vi "VMI_camera_Set.vi"(8 "error in (no error)":errorcluster, 10 "Camera Settings":T1={"Run Options"=1, "Run Mode"=0, "Attributes"="[NIIMAQ_HEADER]\nType = 2\nVersion = 8\n\n[CAMERA_DATA]\nAcquisitionAttributes::VideoMode = \"640 x 480 Mono 8 60.00 fps\"\nAcquisitionAttributes::OffsetX = \"0\"\nAcquisitionAttributes::OffsetY = \"0\"\nAcquisitionAttributes::Width = \"640\"\nAcquisitionAttributes::Height = \"480\"\nAcquisitionAttributes::Bayer::Algorithm = \"Bilinear\"\nAcquisitionAttributes::Bayer::GainB = \"1\"\nAcquisitionAttributes::Bayer::GainG = \"1\"\nAcquisitionAttributes::Bayer::GainR = \"1\"\nAcquisitionAttributes::Bayer::Pattern = \"Use hardware value\"\nAcquisitionAttributes::BitsPerPixel = \"Use hardware value\"\nAcquisitionAttributes::Controller::DesiredStreamChannel = \"0\"\nAcquisitionAttributes::Controller::StreamChannelMode = \"Automatic\"\nAcquisitionAttributes::IgnoreFirstFrame = \"false\"\nAcquisitionAttributes::ImageDecoderCopyMode = \"Auto\"\nAcquisitionAttributes::OutputImageType = \"Auto\"\nAcquisitionAttributes::OverwriteMode = \"Get Newest\"\nAcquisitionAttributes::PixelSignedness = \"Signed\"\nAcquisitionAttributes::ReceiveTimestampMode = \"None\"\nAcquisitionAttributes::ReserveDualPackets = \"false\"\nAcquisitionAttributes::ShiftPixelBits = \"false\"\nAcquisitionAttributes::Speed = \"400 Mbps\"\nAcquisitionAttributes::SwapPixelBytes = \"false\"\nAcquisitionAttributes::Timeout = \"5000\"\nCameraAttributes::Brightness::Mode = \"Relative\"\nCameraAttributes::Gain::Mode = \"Relative\"\nCameraAttributes::Shutter::Mode = \"Relative\"\nCameraAttributes::Brightness::Value = \"16\"\nCameraAttributes::Gain::Value = \"450\"\nCameraAttributes::Shutter::Value = \"700\"\nCameraAttributes::Trigger::TriggerMode = \"Off\"\nCameraAttributes::Trigger::TriggerActivation = \"Level High\"\nCameraAttributes::Trigger::TriggerSource = \"Source 0\"\n", "Peak Find Settings"={"Objects"=0, "Threshold"=128, "Reject Border"=FALSE, "Fill Holes"=FALSE, "Min Object Size"=FALSE, "Min Size"=3, "Max Object Size"=FALSE, "Max Size"=100, "Show Search Area"=FALSE, "Show Center"=FALSE, "Show Bounding Box"=FALSE}, "Image Type"=0, "Test Image File Path"=path "C:/Users/Parkes/Documents/GitHub/Camera-Acquire_Labview/mcp_hit_test.png", "Camera Name"="cam0", "X Size"=640.0, "Y Size"=480.0} {"Image Type" items=["Grayscale (U8)", "Grayscale (I16)", "Grayscale (SGL)", "Complex (CSG)", "RGB (U32)", "HSL (U32)", "RGB (U64)", "Grayscale (U16)"]; "Peak Find Settings"."Objects" items=["Bright Objects", "Dark Objects"]; "Peak Find Settings"."Threshold" min=1 max=999999999 step=1; "Peak Find Settings"."Max Size" min=1 max=999999999 step=1; "Peak Find Settings"."Min Size" min=1 max=999999999 step=1; "Run Mode" items=["Simple Collect", "Collect Images", "Delay Scan"]; "Run Options" items=["Collect Camera", "Test with Image"]}) -> (0 "error out":errorcluster, 2 "Session Out":T3, 3 "Refnum out":T4)   [LabVIEW 2019]
uses:
  <vilib>/vision/Image Controls.llb/IMAQ Image.ctl
  <vilib>/userDefined/High Color/IMAQdx.ctl
  Type defs/VMI_camera_contrl.ctl
  <vilib>/vision/driver/NI_Vision_Acquisition_Software.lvlib
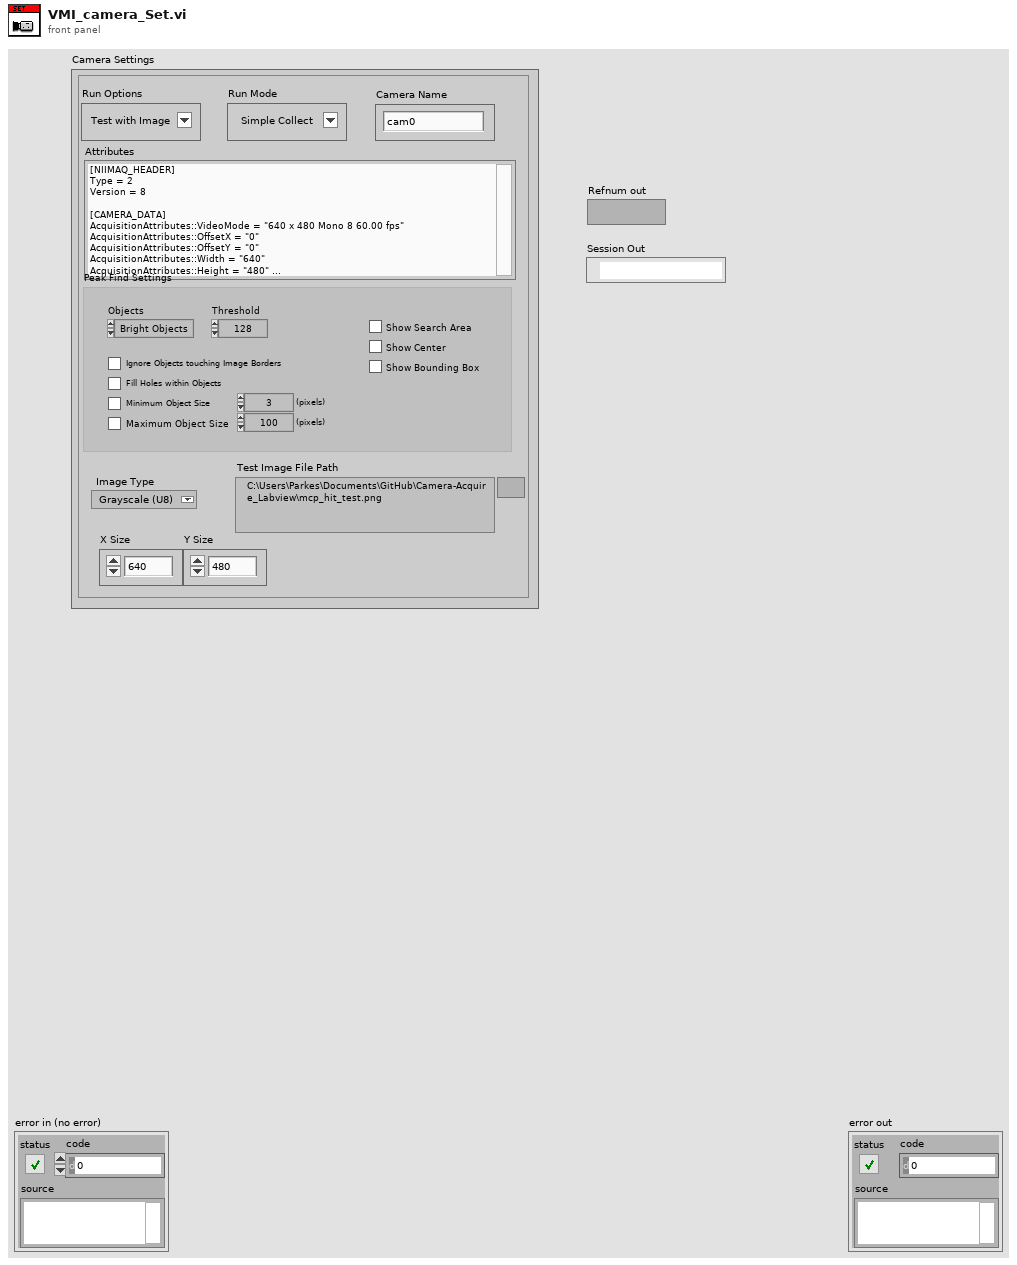
[diagram p1: front panel]
types:
  T1 = typedef "VMI_camera_contrl.ctl" = cluster{"Run Options":u16, "Run Mode":u16, "Attributes":string, "Peak Find Settings":cluster{"Objects":u16, "Threshold":i32, "Reject Border":bool, "Fill Holes":bool, "Min Object Size":bool, "Min Size":i32, "Max Object Size":bool, "Max Size":i32, "Show Search Area":bool, "Show Center":bool, "Show Bounding Box":bool}, "Image Type":T2, "Test Image File Path":path, "Camera Name":string, "X Size":dbl, "Y Size":dbl}
  T2 = typedef "Image Type" = u32
  T3 = typedef "IMAQdx.ctl" = refnum<k21>
  T4 = typedef "IMAQ Image.ctl" = refnum<image>
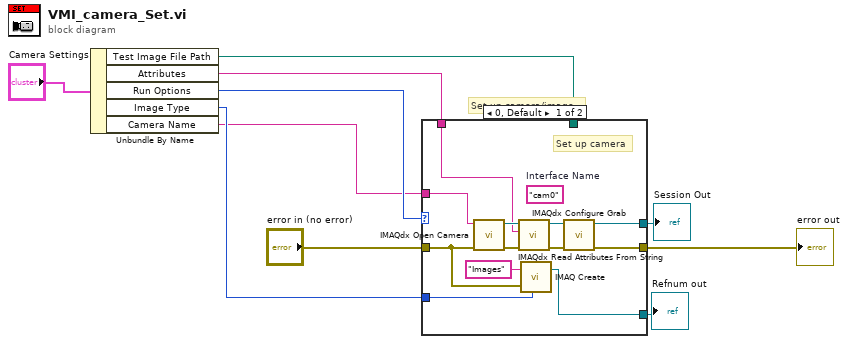
[diagram p0: block diagram]
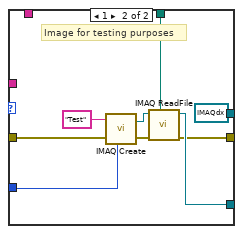
[diagram p2: hidden frame]
diagram:
  # "Set up camera/image"
  n1 = Unbundle By Name("Camera Settings") -> ("Test Image File Path"=w3:path, "Attributes"=w4:string, "Run Options"=w5:u16, "Image Type"=w2:T2, "Camera Name"=w1:string)
  n2 = case shown="0, Default" w5 {
    tunnel: [w15 w28] -> w7
    tunnel: "error in (no error)" -> [w17 w27]
    tunnel: [w20 w26] -> w9
    tunnel: [w14 T3 refnum ("Session Out")] -> w8
    tunnel: w4 -> [w13 _]
    tunnel: w3 -> [_ w24]
    tunnel: w2 -> [w12 w23]
    tunnel: w1 -> [w11 _]
    frame 0, Default {
      (unwired) "cam0"  # Interface Name
      # "Set up camera"
      n3 = call <vilib>:"IMAQdx Open Camera.vi"("error in"=w17, "Session In"=w11) -> ("error out"=w22:errorcluster, "Session Out"=w18:T3)  [unwired: 1 in, 7 out]
      n4 = call <vilib>:"IMAQdx Read Attributes From String.vi"("error in"=w22, "Attributes String In"=w13, "Session In"=w18) -> ("error out"=w21:errorcluster, "Session Out"=w19:T3)  [unwired: 7 out]
      n5 = call "IMAQ Create"("Image Name"="Images", "Image Type"=w12, "error in (no error)"=w17) -> ("New Image"=w15:T4)  [unwired: 2 in, 1 out]
      n6 = call <vilib>:"IMAQdx Configure Grab.vi"("error in"=w21, "Session In"=w19) -> ("error out"=w20:errorcluster, "Session Out"=w14:T3)  [unwired: 1 in, 7 out]
    }
    frame 1 {
      # "Image for testing purposes"
      n7 = call "IMAQ Create"("Image Name"="Test", "Image Type"=w23, "error in (no error)"=w27) -> ("New Image"=w30:T4, "error out"=w29:errorcluster)  [unwired: 2 in]
      n8 = call "IMAQ ReadFile"("File Path"=w24, "error in (no error)"=w29, "Image"=w30) -> ("error out"=w26:errorcluster, "Image Out"=w28:T4)  [unwired: 4 in, 3 out]
    }
  }
  "Refnum out" <- w7
  "Session Out" <- w8
  "error out" <- w9
